vi "Laser 1 Initialise L3.vi"(7 "Independent?":bool, 8 "Error in":errorcluster caption="Error in (no error)", 9 "Wavelength (set) [nm]":u16, 10 "PreChrp1 \nVisa resource":T1, 11 "Ls1 Visa \nresource":T1) -> (0 "Error out":errorcluster)   [LabVIEW 2020]
uses:
  Serial Comms/Visa resource.ctl
  Type Defs/Ls1 Operations.ctl
  Type Defs/Ls1 User Ops.ctl
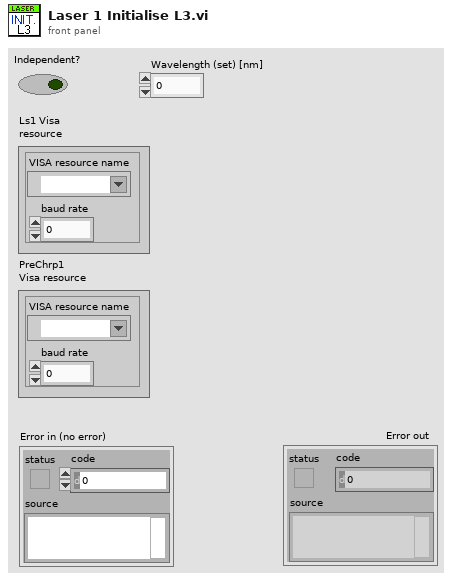
[diagram p1: front panel]
types:
  T1 = typedef "Visa resource.ctl" = cluster{"VISA resource name":refnum<visa-resource-name>, "baud rate":u32}
  T2 = typedef "Ls1 User Ops.ctl" = enum16{"Setup", "Initialise", "Disable Controls", "Enable Controls", "Update Connection Info", "Update Laser Warning", "Update Laser status", "Update Laser status - sel", "Update Laser Wav.", "Update Laser Power", "Update prechiper settings", "Update Laser Note", "Update Shutter Status", "Close"}
  T3 = typedef "Ls1 Operations.ctl" = enum16{"Initialise Connections", "Initialise system", "Check Status", "Open/Close Shutter", "Start/Stop Pump Peak Hold", "Set wavelength", "Close"}
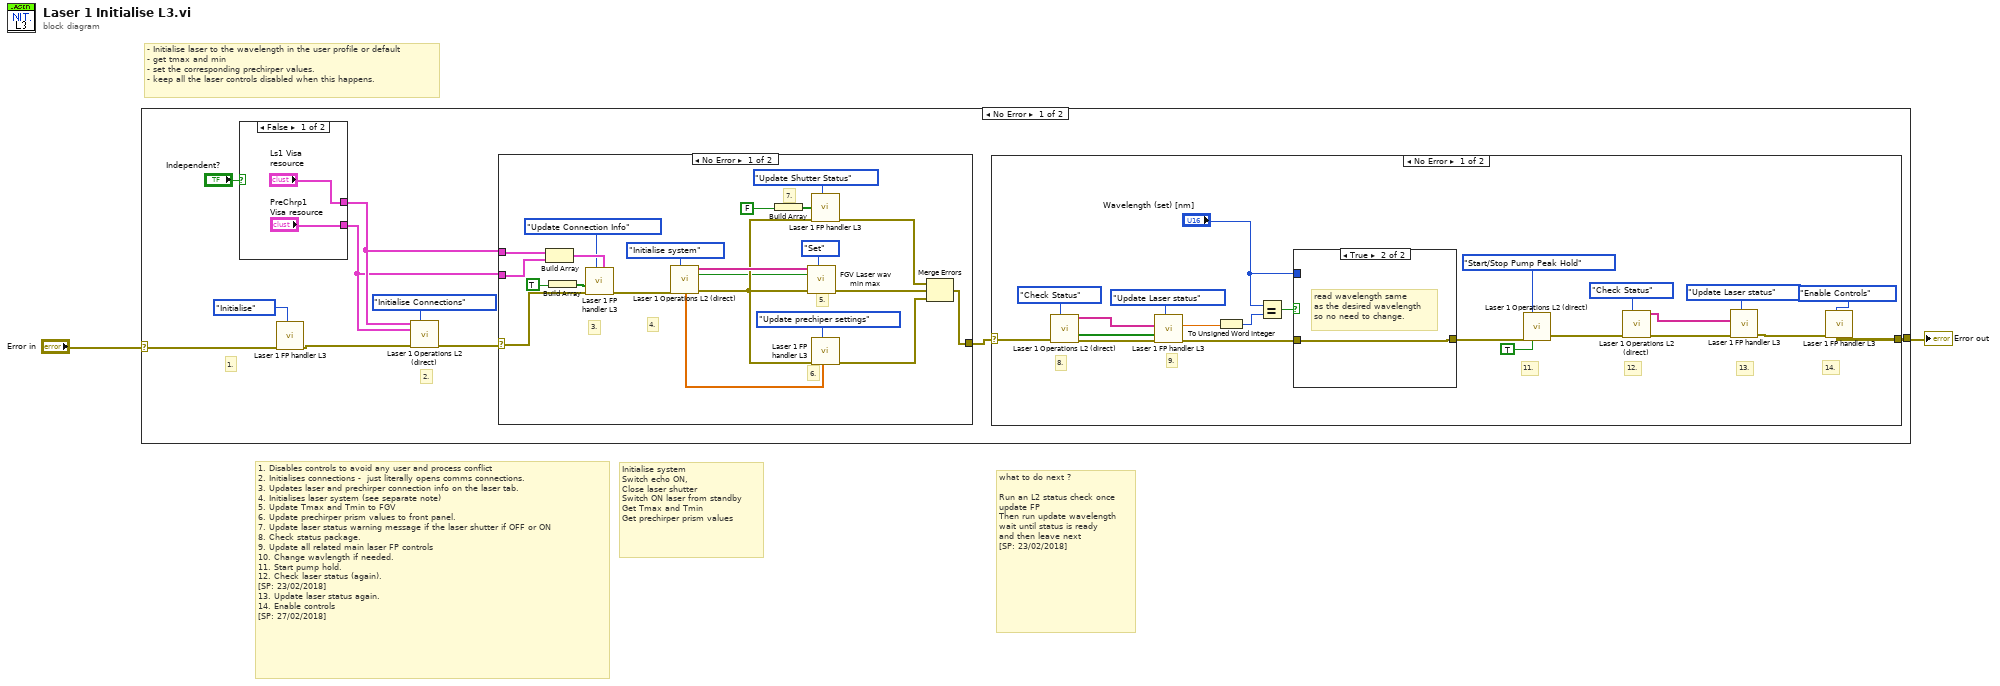
[diagram p0: block diagram]
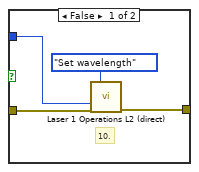
[diagram p2: hidden frame]
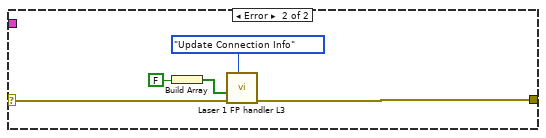
[diagram p4: hidden frame]
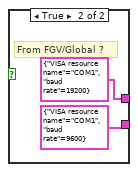
[diagram p5: hidden frame]
diagram:
  # "what to do next ?\n\nRun an L2 status check once\nupdate FP\nThen run update wavelength\nwait until status is ready\nand then leave next\n[SP: 23/02/2018]"
  # "Initialise system\nSwitch echo ON,\nClose laser shutter\nSwitch ON laser from standby\nGet Tmax and Tmin\nGet prechirper prism values"
  # "1. Disables controls to avoid any user and process conflict\n2. Initialises connections -  just literally opens comms connections.\n3. Updates laser and prechirper connection info on the laser tab.\n4. Initialises laser system (see separate note)\n5. Update Tmax and Tmin to FGV\n6. Update prechirper prism values to front panel.\n7. Update laser status warning message if the laser shutter if OFF or ON\n8. Check status package. \n9. Update all related main laser FP controls\n10. Change wavlength if needed.\n11. Start pump hold.\n12. Check laser status (again).\n[SP: 23/02/2018]\n13. Update laser status again.\n14. Enable controls\n[SP: 27/02/2018]"
  # "- Initialise laser to the wavelength in the user profile or default\n- get tmax and min\n- set the corresponding prechirper values.\n- keep all the laser controls disabled when this happens."
  n1 = case shown="No Error" "Error in" {
    selector: "Error in" -> [w3 w72]
    tunnel: [w7 w72] -> w1
    frame No Error {
      # "2."
      # "1."
      n2 = case shown="False" "Independent?" {
        tunnel: ["Ls1 Visa \nresource" T1 {"VISA resource name"="COM1", "baud rate"=19200} ("Ls1 Visa \nresource")] -> w10
        tunnel: ["PreChrp1 \nVisa resource" T1 {"VISA resource name"="COM1", "baud rate"=9600} ("PreChrp1 \nVisa resource")] -> w9
        frame False {
        }
        frame True {
          # "From FGV/Global ?"
        }
      }
      n3 = call "Laser 1 FP handler L3.vi"("FP Ops"=Ls1_User_Ops."Initialise", "Error in"=w3) -> ("Error out"=w4:errorcluster)  [unwired: 7 in, 2 out]
      n4 = call "Laser 1 Operations L2 (direct).vi"("Ls1 Visa \nresource"=w10, "Laser Ops\n actions"=Ls1_Operations."Initialise Connections" ("Laser Ops\n actions"), "PreChrp1 \nVisa resource"=w9, "error in (no error)"=w4) -> ("error out"=w11:errorcluster)  [unwired: 6 in, 5 out]
      n5 = case shown="No Error" w11 {
        selector: w11 -> [w59 w67]
        tunnel: w10 -> [w62 _]
        tunnel: w9 -> [w61 _]
        tunnel: [w49 w66] -> w8
        frame No Error {
          # "7."
          # "6."
          # "5."
          # "4."
          # "3."
          n6 = Build Array(w62, w61) -> (w60:T1[])
          n7 = Build Array(TRUE ("Boolean")) -> (w45:bool[])
          n8 = call "Laser 1 FP handler L3.vi"("VISA Resource"=w60, "FP Ops"=Ls1_User_Ops."Update Connection Info", "Error in"=w59, "Boolean"=w45) -> ("Error out"=w56:errorcluster)  [unwired: 5 in, 2 out]
          n9 = call "Laser 1 Operations L2 (direct).vi"("Laser Ops\n actions"=Ls1_Operations."Initialise system" ("Laser Ops\n actions"), "error in (no error)"=w56) -> ("Ls Data"=w52:string[], "Resp Validated"=w41:bool, "prism Values"=w53:dbl[], "error out"=w51:errorcluster)  [unwired: 8 in, 2 out]
          n10 = Build Array(FALSE) -> (w42:bool[])
          n11 = call "FGV Laser wav min max.vi"("FGV Actions"=enum16{"Get", "Set"}."Set", "error in (no error)"=w51, "Resp Validated?"=w41, "T values"=w52) -> ("error out"=w55:errorcluster)  [unwired: 5 in, 2 out]
          n12 = call "Laser 1 FP handler L3.vi"("FP Ops"=Ls1_User_Ops."Update Shutter Status", "Error in"=w51, "Boolean"=w42) -> ("Error out"=w50:errorcluster)  [unwired: 6 in, 2 out]
          n13 = call "Laser 1 FP handler L3.vi"("Numeric"=w53, "FP Ops"=Ls1_User_Ops."Update prechiper settings", "Error in"=w51) -> ("Error out"=w54:errorcluster)  [unwired: 6 in, 2 out]
          n14 = Merge Errors(w50, w55, w54) -> (w49:errorcluster)
        }
        frame Error {
          n15 = Build Array(FALSE ("Boolean")) -> (w63:bool[])
          n16 = call "Laser 1 FP handler L3.vi"("FP Ops"=Ls1_User_Ops."Update Connection Info", "Error in"=w67, "Boolean"=w63) -> ("Error out"=w66:errorcluster)  [unwired: 6 in, 2 out]
        }
      }
      n17 = case shown="No Error" w8 {
        selector: w8 -> [w34 w40]
        tunnel: [w14 w40] -> w7
        frame No Error {
          # "14."
          # "13."
          # "12."
          # "11."
          # "9."
          # "8."
          n18 = call "Laser 1 Operations L2 (direct).vi"("Laser Ops\n actions"=Ls1_Operations."Check Status" ("Laser Ops\n actions"), "error in (no error)"=w34) -> ("Ls Data"=w30:string[], "Resp Validated (array) ?"=w29:bool[], "error out"=w32:errorcluster)  [unwired: 8 in, 3 out]
          n19 = call "Laser 1 FP handler L3.vi"("FP Ops"=Ls1_User_Ops."Update Laser status", "Error in"=w32, "Boolean"=w29, "I/p string(s)"=w30) -> ("Error out"=w28:errorcluster, "Read Wavelength"=w27:dbl)  [unwired: 5 in, 1 out]
          n20 = To Unsigned Word Integer(number=w27) -> (unsigned 16bit integer=w26:u16)
          n21 = Equal?(x="Wavelength (set) [nm]", y=w26) -> (x = y?=w24:bool)
          n22 = case shown="True" w24 {
            tunnel: [w37 w39] -> w23
            tunnel: w28 -> [w36 w39]
            tunnel: "Wavelength (set) [nm]" -> [w35 _]
            frame False {
              # "10."
              n23 = call "Laser 1 Operations L2 (direct).vi"("Laser Ops\n actions"=Ls1_Operations."Set wavelength" ("Laser Ops\n actions"), "Wavelength \n(set) [nm]"=w35, "error in (no error)"=w36) -> ("error out"=w37:errorcluster)  [unwired: 7 in, 5 out]
            }
            frame True {
              # "read wavelength same\nas the desired wavelength\nso no need to change."
            }
          }
          n24 = call "Laser 1 Operations L2 (direct).vi"("Laser Ops\n actions"=Ls1_Operations."Start/Stop Pump Peak Hold" ("Laser Ops\n actions"), "error in (no error)"=w23, "Boolean I/P"=TRUE) -> ("error out"=w18:errorcluster)  [unwired: 7 in, 5 out]
          n25 = call "Laser 1 Operations L2 (direct).vi"("Laser Ops\n actions"=Ls1_Operations."Check Status" ("Laser Ops\n actions"), "error in (no error)"=w18) -> ("Ls Data"=w13:string[], "error out"=w17:errorcluster)  [unwired: 8 in, 4 out]
          n26 = call "Laser 1 FP handler L3.vi"("FP Ops"=Ls1_User_Ops."Update Laser status", "Error in"=w17, "I/p string(s)"=w13) -> ("Error out"=w15:errorcluster)  [unwired: 6 in, 2 out]
          n27 = call "Laser 1 FP handler L3.vi"("FP Ops"=Ls1_User_Ops."Enable Controls", "Error in"=w15) -> ("Error out"=w14:errorcluster)  [unwired: 7 in, 2 out]
        }
        frame Error {
        }
      }
    }
    frame Error {
    }
  }
  "Error out" <- w1
